vi "WriteSDO_S16.vi"(4 "SubIndex":i32 format="%x", 6 "Index":i32 format="%x", 7 "nodeID":i32, 8 "error in (no error)":errorcluster, 9 "Instrument Ref In":refnum<k24>) -> (2 "error out":errorcluster, 3 "Instrument Ref Out":refnum<k24>)   [LabVIEW 2019]
uses:
  C:/Users/patrick/Documents/GitHub/levylabpitt/PPMS-Monitor-and-Control/lvsrc/drivers/QDInstrument_LabView/QDInstrument.dll
  QDInstrument.dll
panel:
  in  "writeValue":i16
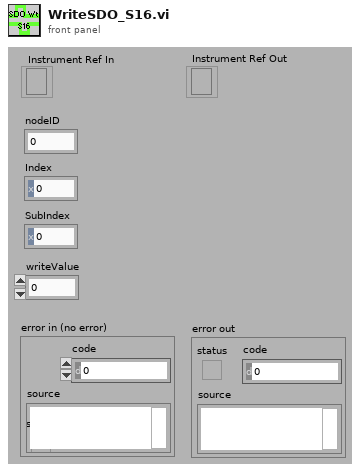
[diagram p1: front panel]
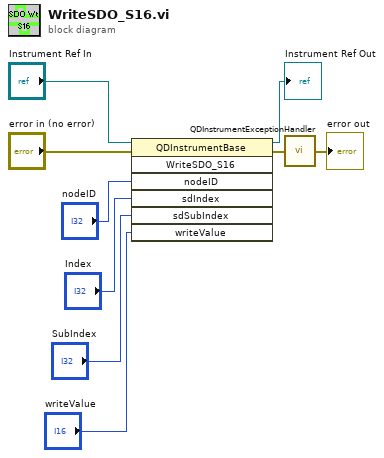
[diagram p0: block diagram]
diagram:
  n1 = invoke class="QDInstrumentBase" method="WriteSDO_S16"(reference="Instrument Ref In", error in="error in (no error)", "nodeID"="nodeID", "sdIndex"="Index", "sdSubIndex"="SubIndex", "writeValue"="writeValue") -> (reference out=→"Instrument Ref Out":refnum<k24>, error out=w3:errorcluster)  [unwired: 1 in, 5 out]
  n2 = call "QDInstrumentExceptionHandler.vi"("Error in"=w3) -> ("Error out"=→"error out":errorcluster)
